vi "chaosui-crest-open.vi"(11 "chaoswanurl":string) -> (3 "handle":T2)   [LabVIEW 2014, in "chaosui-crest.lvlib"]
doc: "chaos_crest_handle_t chaos_crest_open(const char* chaoswanurl);"
uses:
  chaosui-crest.lvlib
  <vilib>/httpClient/ClientHandle.ctl
  <vilib>/httpClient/LabVIEWHTTPClient.lvlib
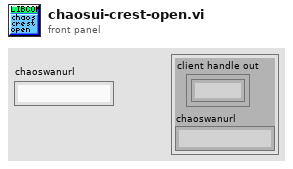
[diagram p1: front panel]
types:
  T1 = typedef "LabVIEWHTTPClient.lvlib/ClientHandle.ctl" = refnum<k1>
  T2 = cluster{"client handle out":T1, "chaoswanurl":string}
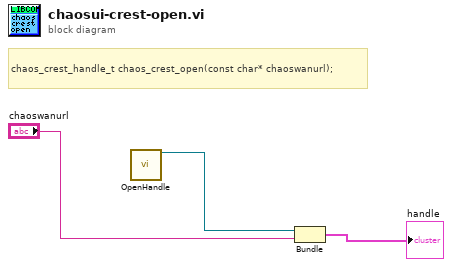
[diagram p0: block diagram]
diagram:
  # "chaos_crest_handle_t chaos_crest_open(const char* chaoswanurl);"
  n1 = call <vilib>:"OpenHandle.vi"() -> ("client handle out"=w2:T1)  [unwired: 14 in, 1 out]
  n2 = Bundle("client handle out"=w2, "chaoswanurl"="chaoswanurl") -> (→"handle":T2)  [unwired: 1 in]
